vi "Save As.vi"(8 "error in (no error)":errorcluster, 9 "File Path Control":path, 10 "File refnum":refnum<k7>) -> (0 "error out":errorcluster, 2 "reference out":refnum<k7>)   [LabVIEW 2020, in "lvpptx.lvlib"]
uses:
  lvpptx.lvlib
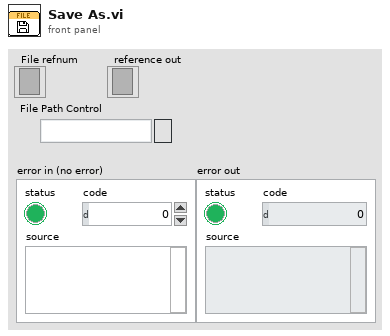
[diagram p1: front panel]
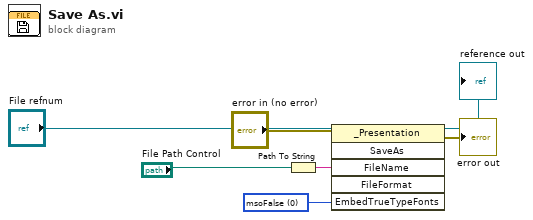
[diagram p0: block diagram]
diagram:
  w6 = 0 items=["msoTrue"=-1, "msoFalse"=0, "msoCTrue"=1, "msoTriStateToggle"=-3, "msoTriStateMixed"=-2] ("EmbedTrueTypeFonts")
  n1 = Path To String(path="File Path Control") -> (string=w5:string)
  n2 = invoke class="_Presentation" method="SaveAs"(reference="File refnum", error in="error in (no error)", "FileName"=w5, "EmbedTrueTypeFonts"=w6) -> (reference out=→"reference out":refnum<k7>, error out=→"error out":errorcluster)  [unwired: 2 in, 4 out]
